vi "Enqueue Analog Output Command.vi"(10 "Analog Output Command":T1 {"State" scale=0.0..5.0}, 11 "Queue In":refnum<queue>) -> ()   [LabVIEW 2020]
uses:
  Type Definitions/Analog Output Command.ctl
  Type Definitions/Payload Class.ctl
  Type Definitions/Enum - Commands.ctl
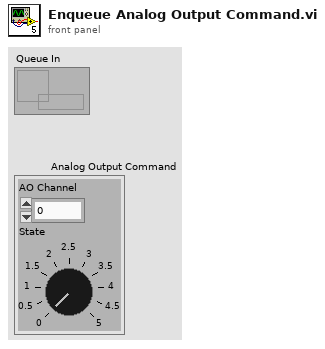
[diagram p1: front panel]
types:
  T1 = typedef "Analog Output Command.ctl" = cluster{"AO Channel":u8, "State":dbl}
  T2 = typedef "Enum - Commands.ctl" = enum16{"Null", "Analog Output Command", "Digital Output Command"}
  T3 = typedef "Payload Class.ctl" = enum16{"System State", "Parameters", "Metadata", "Software Monitor", "Data", "Commands"}
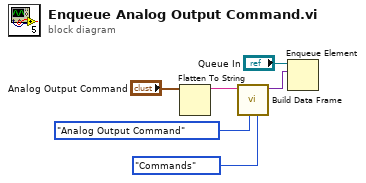
[diagram p0: block diagram]
diagram:
  n1 = Flatten To String(anything="Analog Output Command") -> (data string=w6:string)  [unwired: 3 in, 2 out]
  n2 = call "Build Data Frame.vi"("Payload Class (Data)"=Payload_Class."Commands", "Payload ID (0)"=Enum_-_Commands."Analog Output Command" ("Commands"), "Payload (Empty String)"=w6) -> ("Frame"=w3:variant)  [unwired: 7 in, 1 out]
  n3 = Enqueue Element(queue="Queue In", element=w3) -> ()  [unwired: 2 in, 3 out]
